vi "DAQtesk.vi"(8 "error in":errorcluster) -> (0 "error out":errorcluster, 3 "task out":refnum<k21>)   [LabVIEW 2016]
uses:
  <vilib>/DAQmx/configure/timing.llb/DAQmx Timing (Sample Clock).vi
  <vilib>/DAQmx/create/channels.llb/DAQmx Create Channel (AI-Temperature-Thermocouple).vi
  <vilib>/DAQmx/create/channels.llb/DAQmx Create Channel (AI-Voltage-Basic).vi
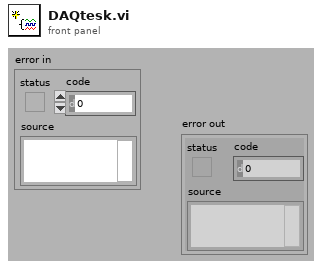
[diagram p1: front panel]
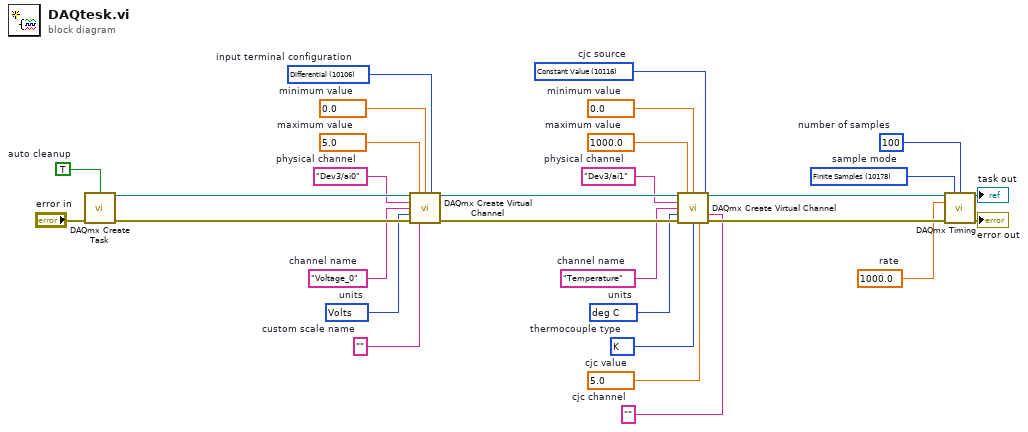
[diagram p0: block diagram]
diagram:
  w1 = 10178 items=["Finite Samples"=10178, "Continuous Samples"=10123, "Hardware Timed Single Point"=12522]  # sample mode
  w2 = 100  # number of samples
  w3 = 1000.0  # rate
  w7 = 10116 items=["Built-In"=10200, "Constant Value"=10116, "Channel"=10113]  # cjc source
  w9 = ""  # cjc channel
  w10 = 5.0  # cjc value
  w11 = 10073 items=["J"=10072, "K"=10073, "N"=10077, "R"=10082, "S"=10085, "T"=10086, "B"=10047, "E"=10055]  # thermocouple type
  w12 = 10143 items=["deg C"=10143, "deg F"=10144, "Kelvins"=10325, "deg R"=10145, "From Custom Scale"=10065]  # units
  w8 = "Temperature"  # channel name
  w14 = 0.0  # minimum value
  w15 = 1000.0  # maximum value
  w16 = "Dev3/ai1"  # physical channel
  w18 = 10106 items=["default"=-1, "RSE"=10083, "NRSE"=10078, "Differential"=10106, "Pseudodifferential"=12529]  # input terminal configuration
  w19 = 10348 items=["Volts"=10348, "From Custom Scale"=10065]  # units
  w20 = "Voltage_0"  # channel name
  w22 = ""  # custom scale name
  w23 = 0.0  # minimum value
  w24 = 5.0  # maximum value
  w25 = "Dev3/ai0"  # physical channel
  w27 = TRUE  # auto cleanup
  n1 = call <vilib>:"DAQmx Create Task.vi"("auto cleanup"=w27, "error in"="error in") -> ("task out"=w26:refnum<k21>, "error out"=w28:errorcluster)  [unwired: 12 in]
  n2 = call-poly <vilib>:"DAQmx Create Virtual Channel.vi"("task in"=w26, "maximum value"=w24, "minimum value"=w23, "input terminal configuration"=w18, "physical channels"=w25, "name to assign"=w20, "units"=w19, "error in"=w28, "custom scale name"=w22) -> ("task out"=w17:refnum<k21>, "error out"=w21:errorcluster)  [unwired: 5 in]
  n3 = call-poly <vilib>:"DAQmx Create Virtual Channel.vi"("task in"=w17, "maximum value"=w15, "minimum value"=w14, "physical channels"=w16, "cjc source"=w7, "name to assign"=w8, "units"=w12, "cjc channel"=w9, "error in"=w21, "thermocouple type"=w11, "cjc value"=w10) -> ("task out"=w4:refnum<k21>, "error out"=w13:errorcluster)  [unwired: 3 in]
  n4 = call-poly <vilib>:"DAQmx Timing.vi"("task/channels in"=w4, "sample mode"=w1, "samples per channel"=w2, "rate"=w3, "error in"=w13) -> ("task out"=→"task out":refnum<k21>, "error out"=→"error out":errorcluster)  [unwired: 9 in]
